vi "Default Instrument Setup.vi"(8 "error in (no error)":errorcluster, 11 "VISA resource name":refnum<visa-resource-name>) -> (0 "error out":errorcluster, 3 "VISA resource name out":refnum<visa-resource-name>)   [LabVIEW 2020, in "SR830.lvlib"]
doc: "This Utility VI sends a default command string to the instrument whenever a new VISA session is opened, or the instrument is reset. Use this VI as a subVI for the Initialize and Reset VIs. Altering this VI could cause these two VIs to operate incorrectly."
uses:
  SR830.lvlib
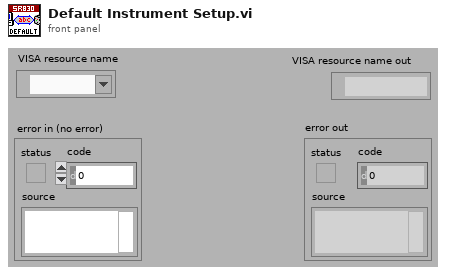
[diagram p1: front panel]
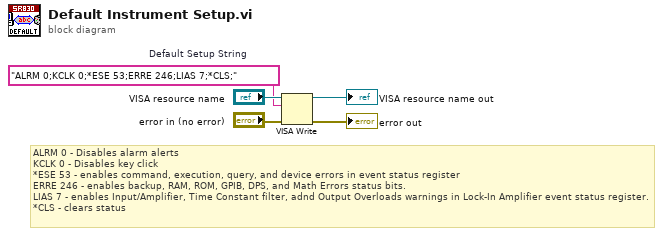
[diagram p0: block diagram]
diagram:
  w1 = "ALRM 0;KCLK 0;*ESE 53;ERRE 246;LIAS 7;*CLS;"  # Default Setup String
  # "ALRM 0 - Disables alarm alerts\nKCLK 0 - Disables key click\n*ESE 53 - enables command, execution, query, and device errors in event status register\nERRE 246 - enables backup, RAM, ROM, GPIB, DPS, and Math Errors status bits.\nLIAS 7 - enables Input/Amplifier, Time Constant filter, adnd Output Overloads warnings in Lock-In Amplifier event status register.\n*CLS - clears status"
  n1 = VISA Write(VISA resource name="VISA resource name", write buffer=w1, error in (no error)="error in (no error)") -> (VISA resource name out=→"VISA resource name out":refnum<visa-resource-name>, error out=→"error out":errorcluster)  [unwired: 1 out]
